vi "PC Benchmarking.vi"(8 "error in":errorcluster, 9 "run time":u32, 10 "target alias":string="PC Benchmarking", 11 "configuration file path":path=path "C:/Users/bsnover/Desktop/DCAF Integration Testing/Testing Project/Integration Testing Configuration.pcfg") -> (0 "error out":errorcluster, 3 "engine status":string)   [LabVIEW 2014]
doc: "This application launches and executes the Tag Bus Data framework configuration for the specified target alias. This is a simple example of the framework API functions, but may also be a suitable starting point for a Host UI or Thick Client that is running a local version of the framework."
uses:
  <vilib>/NI/Module Execution Interface/Engine Runtime/Execution States.ctl
  <vilib>/NI/Module Execution Interface/Engine Runtime/Fault.ctl
  <vilib>/NI/Tag Bus Module Framework/runtime/error classification.ctl
  <vilib>/NI/Module Execution Interface/Engine Runtime/Engine Runtime Interface.lvclass
  <vilib>/NI/DCAF/Tag Editor Core/Framework Configuration Classes/target runtime/PL_Target Runtime.lvclass
  <vilib>/NI/Tag Bus Module Framework/runtime/TBM module execution interface.lvclass
panel:
  out "engine status":T4(array[cluster])
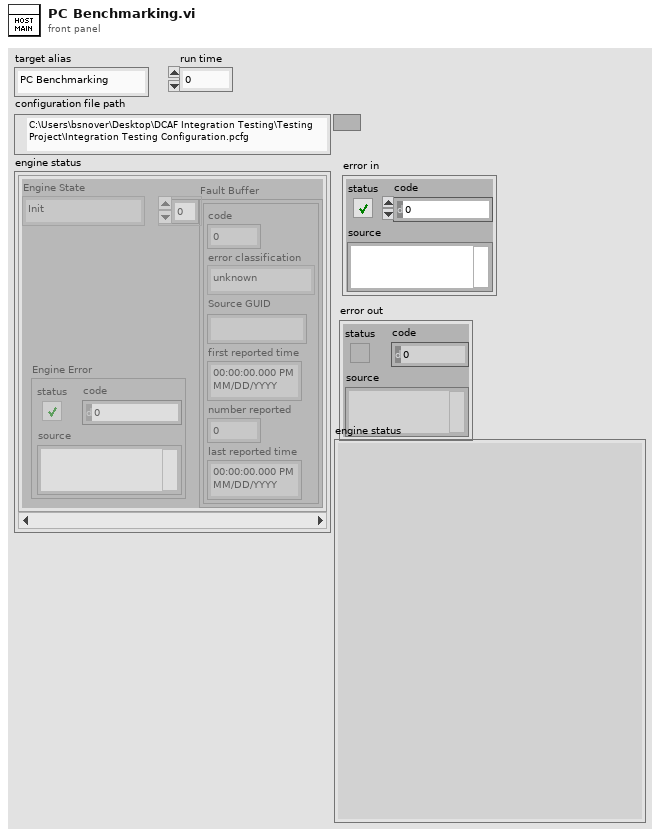
[diagram p1: front panel]
types:
  T1 = typedef "Engine Runtime Interface.lvclass/Execution States.ctl" = enum16{"Init", "Pre-Operational", "Safe-Operational", "Operational", "Stopped"}
  T2 = typedef "Engine Runtime Interface.lvclass/Fault.ctl" = cluster{"code":i32, "error classification":T3, "Source GUID":string, "first reported time":timestamp, "number reported":u32, "last reported time":timestamp}
  T3 = typedef "TBM module execution interface.lvclass/error classification.ctl" = enum16{"unknown", "none", "trivial", "recoverable", "critical"}
  T4 = cluster{"Engine State":T1, "Fault Buffer":T2[], "Engine Error":errorcluster}[]
  T5 = cluster{"Engine State":T1, "faults":T2[], "Engine Error":errorcluster}
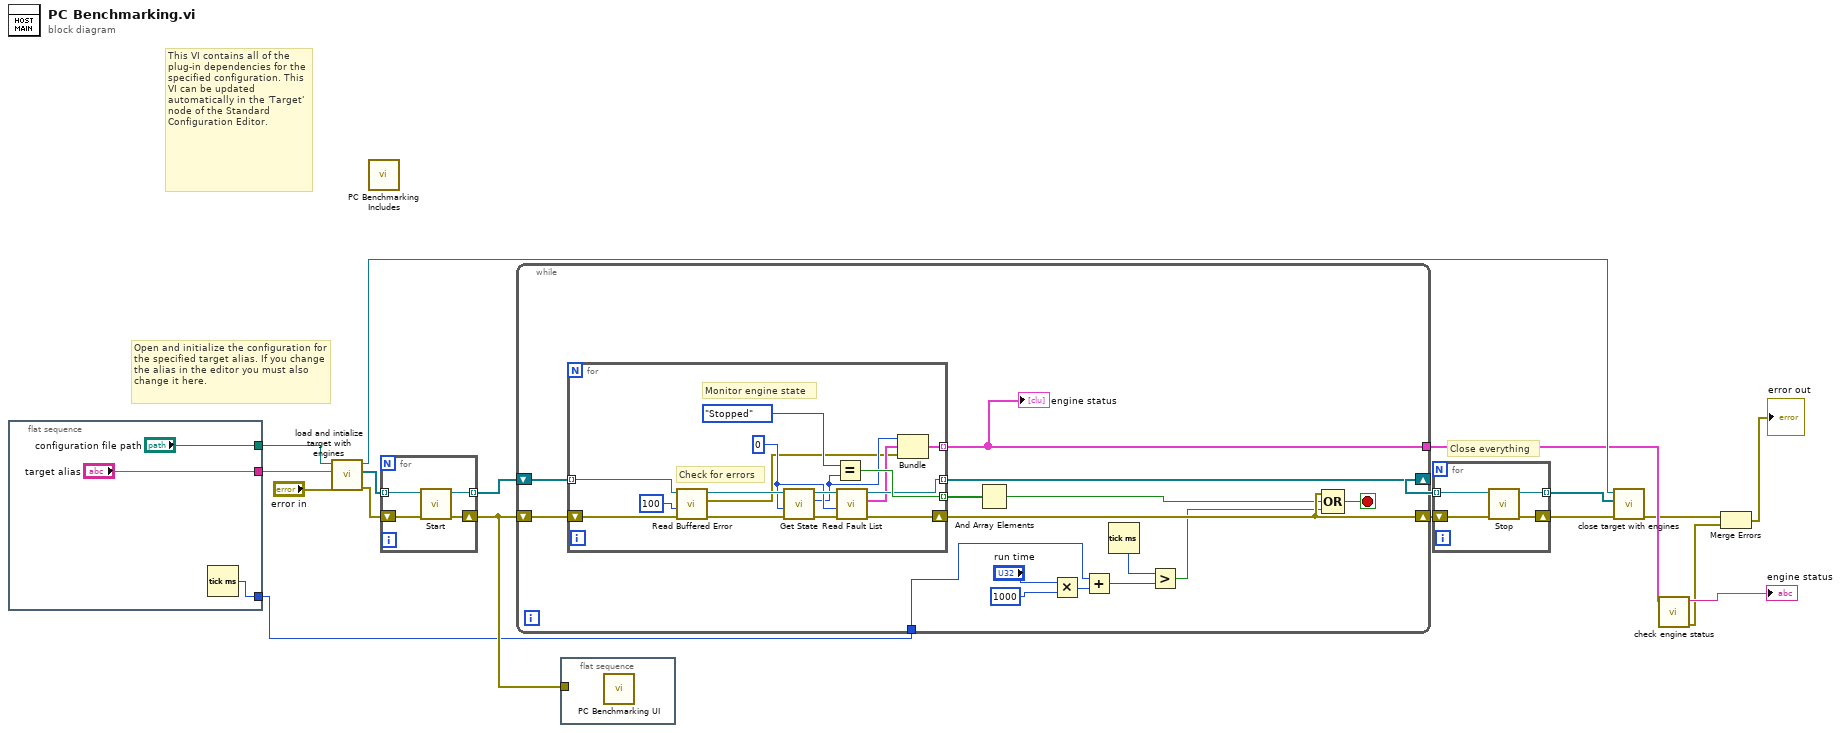
[diagram p0: block diagram]
diagram:
  # "Open and initialize the configuration for the specified target alias. If you change the alias in the editor you must also change it here."
  # "Close everything"
  # "This VI contains all of the plug-in dependencies for the specified configuration. This VI can be updated automatically in the 'Target' node of the Standard Configuration Editor."
  n1 = flat-sequence {
    tunnel: ["target alias"] -> w8
    tunnel: ["configuration file path"] -> w7
    tunnel: [w19] -> w9
    frame #0 {
      n2 = Tick Count (ms)() -> (millisecond timer value=w19:u32)
    }
  }
  n3 = call <vilib>:"load and intialize target with engines.vi"("error in"="error in", "target alias"=w8, "file path"=w7) -> ("error out"=w15:errorcluster, "engine runtime interfaces"=w14:refnum<class "Engine Runtime Interface.lvclass">[], "target runtime"=w12:refnum<class "PL_Target Runtime.lvclass">)  [unwired: 6 in]
  n4 = call "PC Benchmarking Includes.vi"() -> ()  [unwired: 12 in]
  n5 = for {
    tunnel: [w25] -> w18 mode=indexing
    tunnel: w14 -> [w22] mode=indexing
    shift-right: [w24] -> w10
    shift-left: w15 -> [w23]
    n6 = call-dynamic "Start.vi"("error in"=w23, "Engine Runtime Interface in"=w22) -> ("error out"=w24:errorcluster, "Engine Runtime Interface out"=w25:refnum<class "Engine Runtime Interface.lvclass">)  [unwired: 8 in]
  }
  n7 = while {
    shift-right: [w38] -> w17
    shift-left: w18 -> [w40]
    shift-right: [w36] -> w16
    shift-left: w10 -> [w39]
    tunnel: w9 -> [w28]
    tunnel: [w26] -> w5
    stop <- w37 stop-if-true
    n8 = for {
      tunnel: w40 -> [w56] mode=indexing
      tunnel: [w47] -> w38 mode=indexing
      tunnel: [w51] -> w35 mode=indexing
      shift-right: [w46] -> w36
      shift-left: w39 -> [w55]
      tunnel: [w41] -> w26 mode=indexing
      w45 = 0 ("timeout (-1)")
      # "Monitor engine state"
      # "Check for errors"
      n9 = call-dynamic "Read Buffered Error.vi"("error in"=w55, "timeout in ms (0)"=100, "Engine Runtime Interface in"=w56) -> ("error out"=w53:errorcluster, "Engine Error"=w42:errorcluster, "Engine Runtime Interface out"=w54:refnum<class "Engine Runtime Interface.lvclass">)  [unwired: 6 in]
      n10 = call-dynamic "Get State.vi"("error in"=w53, "timeout (-1)"=w45, "Engine Runtime Interface in"=w54) -> ("error out"=w49:errorcluster, "Engine State"=w44:T1, "Engine Runtime Interface out"=w48:refnum<class "Engine Runtime Interface.lvclass">)  [unwired: 6 in]
      n11 = Equal?(x=Execution_States."Stopped" ("Engine State"), y=w44) -> (x = y?=w51:bool)
      n12 = call-dynamic "Read Fault List.vi"("error in"=w49, "timeout (-1)"=w45, "Engine Runtime Interface in"=w48) -> ("error out"=w46:errorcluster, "faults"=w43:T2[], "Engine Runtime Interface out"=w47:refnum<class "Engine Runtime Interface.lvclass">)  [unwired: 6 in]
      n13 = Bundle("Engine State"=w44, "faults"=w43, "Engine Error"=w42) -> (w41:T5)  [unwired: 1 in]
    }
    "engine status" <- w26
    n14 = And Array Elements(Boolean array=w35) -> (logical AND=w34:bool)
    n15 = Multiply(x="run time", y=u32 1000) -> (x*y=w31:u32)
    n16 = Add(x=w28, y=w31) -> (x+y=w29:u32)
    n17 = Tick Count (ms)() -> (millisecond timer value=w27:u32)
    n18 = Greater?(x=w27, y=w29) -> (0:w30:bool)
    n19 = Compound Arithmetic op=OR(w36, w34, w30) -> (w37:bool)
  }
  n20 = flat-sequence {
    tunnel: w10 -> [_]
    frame #0 {
      n21 = call "PC Benchmarking UI.vi"() -> ()  [unwired: 12 in]
    }
  }
  n22 = for {
    tunnel: w17 -> [w60] mode=indexing
    shift-right: [w57] -> w11
    shift-left: w16 -> [w59]
    tunnel: [w58] -> w13 mode=indexing
    n23 = call-dynamic "Stop.vi"("error in"=w59, "Engine Runtime Interface in"=w60) -> ("error out"=w57:errorcluster, "Engine Runtime Interface out"=w58:refnum<class "Engine Runtime Interface.lvclass">)  [unwired: 8 in]
  }
  n24 = call <vilib>:"close target with engines.vi"("error in"=w11, "Engine Runtime Interfaces"=w13, "Target Runtime"=w12) -> ("error out"=w2:errorcluster)  [unwired: 8 in]
  n25 = call "check engine status.vi"("engine status"=w5) -> ("error out"=w1:errorcluster, "JSON string"=→"engine status":string)  [unwired: 9 in]
  n26 = Merge Errors(w2, w1) -> (→"error out":errorcluster)
